vi "ConfigInstr.vi"(6 "InstrumentName":string, 7 "VisaRessIn":refnum<visa-resource-name>, 8 "error in (no error)":errorcluster caption="entrée d'erreur (pas d'erreur)", 9 "FirstClassInst":bool, 10 "Function":string, 11 "MHData In":refnum<class "MultiHarp150.lvclass"> caption="DNL_LabVIEW Object in") -> (0 "error out":errorcluster caption="sortie d'erreur", 3 "MHData Out":refnum<class "MultiHarp150.lvclass"> caption="DNL_LabVIEW Object out")   [LabVIEW 2019, in "MultiHarp150.lvclass"]
uses:
  MultiHarp150.lvclass
  C:/Programmes Labview/LabScanV1A/DevicesClass/BaseDevice/BaseDevice.lvclass
  MultiHarp150_Func.ctl
  MultiHarp150.lvclass/MultiHarp150.ctl
  BaseDevice/BaseDevice.lvclass/BaseDevice.ctl
  BaseDevice/Accessor/SetShowInstrNm.vi
  BaseDevice/Accessor/SetSaveArrVarPar.vi
  BaseDevice/Accessor/SetInstrParam.vi
panel:
  in  "Class_Func":T1
  out "VisaRessOut":refnum<visa-resource-name>
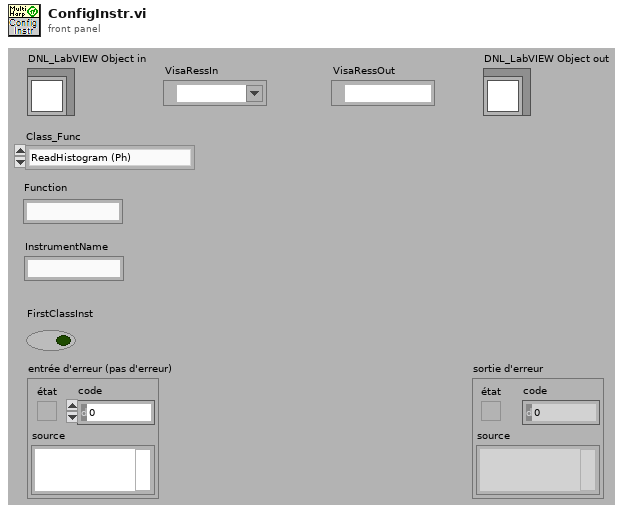
[diagram p1: front panel]
types:
  T1 = typedef "MultiHarp150.lvclass/MultiHarp150_Func.ctl" = enum16{"ReadHistogram (Ph)", "ReadT2 (Ph)", "ReadT3 (Ph)", "ReadCount (Ph)"}
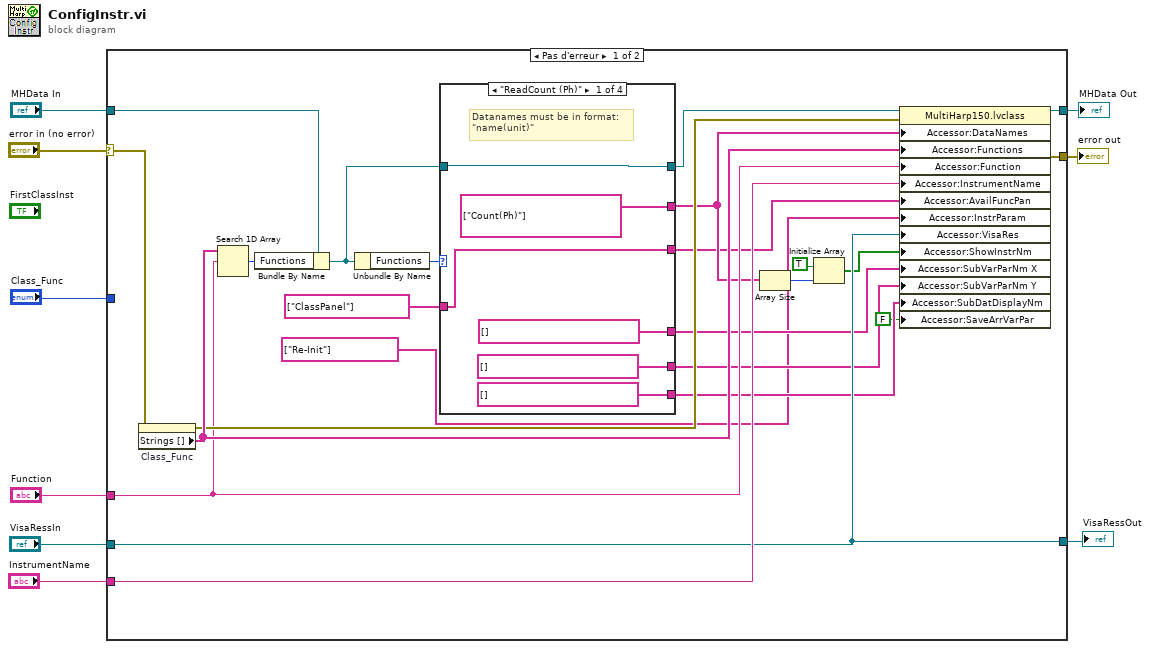
[diagram p0: block diagram]
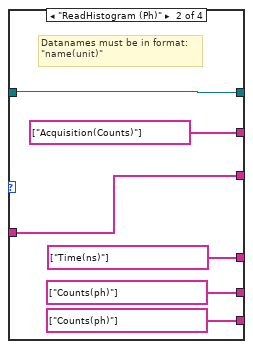
[diagram p2: hidden frame]
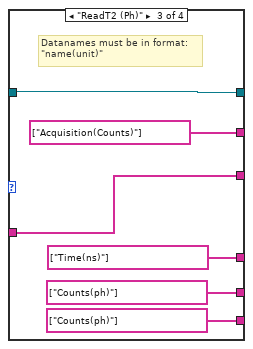
[diagram p3: hidden frame]
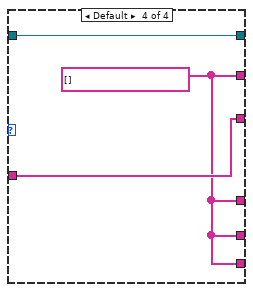
[diagram p4: hidden frame]
diagram:
  n1 = case shown="Pas d'erreur" "error in (no error)" {
    selector: "error in (no error)" -> [w27 w56]
    tunnel: [w33 w56] -> w8
    tunnel: "MHData In" -> [w28 w55]
    tunnel: [w32 w55] -> w6
    tunnel: "Class_Func" -> [_ _]
    tunnel: "Function" -> [w23 _]
    tunnel: "InstrumentName" -> [w22 _]
    tunnel: "VisaRessIn" -> [w21 _]
    tunnel: [w21 _] -> w1
    frame No Error {
      n2 = property on="Class_Func" class="Énum (strict)"(error in=w27) -> (error out=w26:errorcluster, "Strings []"=w30:string[])  [unwired: 1 in, 1 out]
      n3 = Search 1D Array(1D array=w30, element=w23) -> (index of element=w29:i32)  [unwired: 1 in]
      n4 = Bundle By Name(cluster=w28, "Functions"=w29) -> (w25:refnum<class "MultiHarp150.lvclass">)
      n5 = Unbundle By Name(w25) -> ("Functions"=w31:T1)
      n6 = case shown="\"ReadCount (Ph)\"" w31 {
        tunnel: [string[] ["Count(Ph)"] string[] ["Acquisition(Counts)"] string[] ["Acquisition(Counts)"] w52] -> w18
        tunnel: w25 -> [w39 w45 w51 w54]
        tunnel: [w39 w45 w51 w54] -> w24
        tunnel: [w37 w43 w49 w53] -> w15
        tunnel: string[] ["ClassPanel"] -> [w37 w43 w49 w53]
        tunnel: [string[] [] string[] ["Time(ns)"] string[] ["Time(ns)"] w52] -> w14
        tunnel: [string[] [] string[] ["Counts(ph)"] string[] ["Counts(ph)"] w52] -> w13
        tunnel: [string[] [] string[] ["Counts(ph)"] string[] ["Counts(ph)"] w52] -> w12
        frame "ReadCount (Ph)" {
          # "Datanames must be in format:\n\"name(unit)\""
        }
        frame "ReadHistogram (Ph)" {
          # "Datanames must be in format:\n\"name(unit)\""
        }
        frame "ReadT2 (Ph)" {
          # "Datanames must be in format:\n\"name(unit)\""
        }
        frame Default {
          w52 = string[] []
        }
      }
      n7 = Array Size(array=w18) -> (size(s)=w20:i32)
      n8 = Initialize Array(TRUE, w20) -> (w17:bool[])
      n9 = property class="MultiHarp150.lvclass"(reference=w24, error in=w26, "Accessor:DataNames"=w18, "Accessor:Functions"=w30, "Accessor:Function"=w23, "Accessor:InstrumentName"=w22, "Accessor:AvailFuncPan"=w15, "Accessor:InstrParam"=string[] ["Re-Init"], "Accessor:VisaRes"=w21, "Accessor:ShowInstrNm"=w17, "Accessor:SubVarParNm X"=w14, "Accessor:SubVarParNm Y"=w13, "Accessor:SubDatDisplayNm"=w12, "Accessor:SaveArrVarPar"=FALSE ("SaveArrVarPar")) -> (reference out=w32:refnum<class "MultiHarp150.lvclass">, error out=w33:errorcluster)
    }
    frame Error {
    }
  }
  "error out" <- w8
  "MHData Out" <- w6
  "VisaRessOut" <- w1
